vi "ble_read_specific_message.vi"(5 "Command Class (System)":T1 format="%02x" items=["System", "Persistent Store", "Attribute database", "Connection", "Attribute client", "Security Manager", "Generic Access Profile", "Hardware"], 6 "Stop if differnt to expected(F)":bool, 7 "Message Type (Response)":T2 format="%02x" items=["Command / Response"=0, "Event"=128], 8 "error in (no error)":errorcluster, 10 "Message ID (0x00)":u8 format="%02x", 11 "COM Bluegiga in":refnum<visa-resource-name>) -> (0 "error out":errorcluster, 1 "full message package":u8[](array[numeric]) format="%02x", 2 "specific payload":u8[](array[numeric]) format="%02x", 3 "COM Bluegiga out":refnum<visa-resource-name>, 4 "success?":bool)   [LabVIEW 2013]
uses:
  type_def/message_type.ctl
  type_def/message_class.ctl
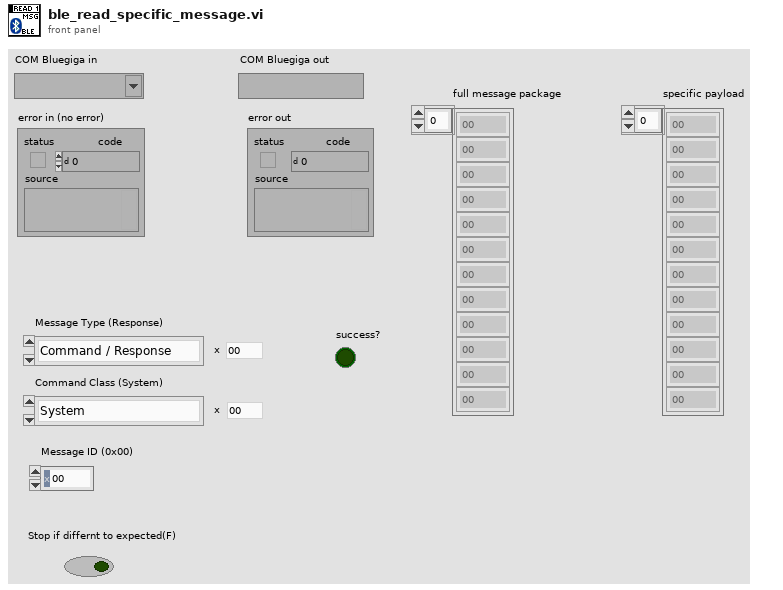
[diagram p1: front panel]
types:
  T1 = typedef "message_class.ctl" = u8
  T2 = typedef "message_type.ctl" = u8
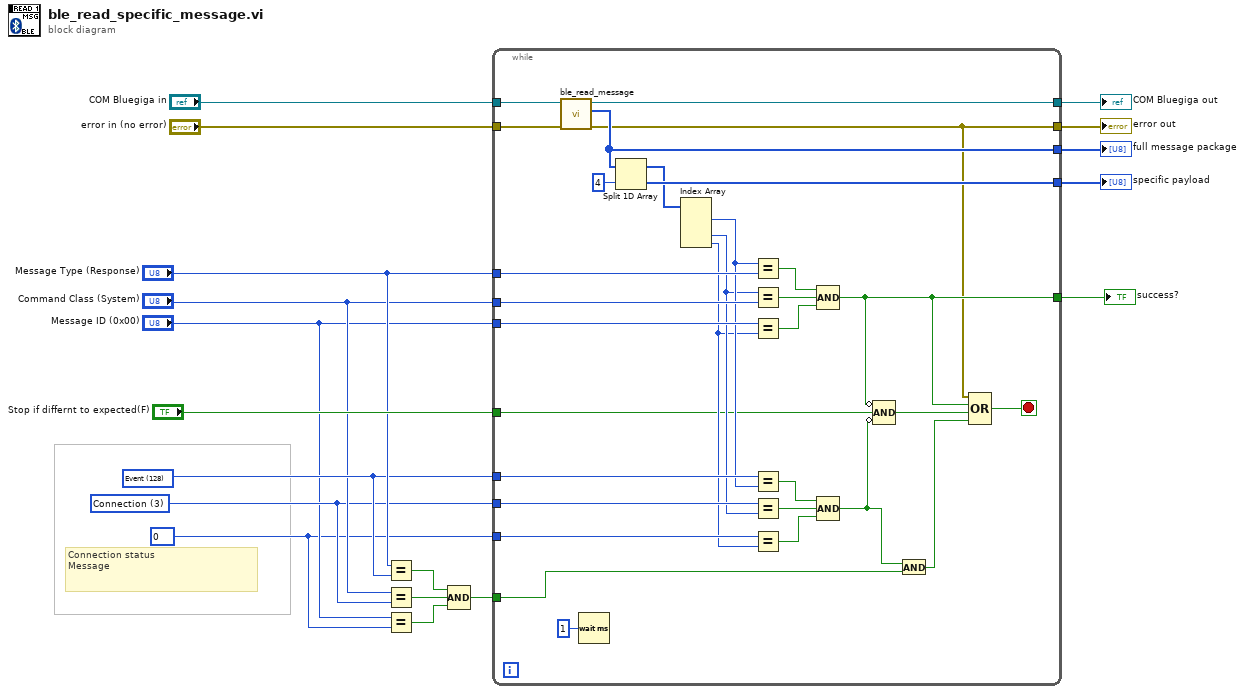
[diagram p0: block diagram]
diagram:
  w5 = u8 0 ("Message ID (0x00)")
  w7 = T1 3 items=["System", "Persistent Store", "Attribute database", "Connection", "Attribute client", "Security Manager", "Generic Access Profile", "Hardware"] ("Command Class (System)")
  w9 = T2 128 items=["Command / Response"=0, "Event"=128] ("Message Type (Response)")
  # "Connection status\nMessage"
  n1 = Equal?(x="Message Type (Response)", y=w9) -> (x = y?=w4:bool)
  n2 = Equal?(x="Command Class (System)", y=w7) -> (x = y?=w3:bool)
  n3 = Equal?(x="Message ID (0x00)", y=w5) -> (x = y?=w2:bool)
  n4 = Compound Arithmetic op=AND(w4, w3, w2) -> (w1:bool)
  n5 = while {
    tunnel: "COM Bluegiga in" -> [w49]
    tunnel: "error in (no error)" -> [w48]
    tunnel: [w47] -> w16
    tunnel: [w19] -> w15
    tunnel: "Message Type (Response)" -> [w46]
    tunnel: "Command Class (System)" -> [w45]
    tunnel: "Message ID (0x00)" -> [w44]
    tunnel: [w43] -> w14
    tunnel: [w42] -> w13
    tunnel: [w26] -> w12
    tunnel: w9 -> [w33]
    tunnel: w7 -> [w32]
    tunnel: w5 -> [w31]
    tunnel: "Stop if differnt to expected(F)" -> [w23]
    tunnel: w1 -> [w21]
    stop <- w22 stop-if-true
    n6 = call "ble_read_message.vi"("error in (no error)"=w48, "COM Bluegiga in"=w49) -> ("error out"=w19:errorcluster, "message package"=w43:u8[], "COM Bluegiga out"=w47:refnum<visa-resource-name>)  [unwired: 7 in]
    n7 = Wait (ms)(milliseconds to wait=u32 1) -> ()  [unwired: 1 out]
    n8 = Split 1D Array(array=w43, index=4) -> (first subarray=w40:u8[], second subarray=w42:u8[])
    n9 = Index Array(array=w40) -> (element #1=w30:u8, element #3=w29:u8, element #4=w28:u8)  [unwired: 4 in, 1 out]
    n10 = Equal?(x=w30, y=w46) -> (x = y?=w39:bool)
    n11 = Equal?(x=w29, y=w45) -> (x = y?=w38:bool)
    n12 = Equal?(x=w44, y=w28) -> (x = y?=w37:bool)
    n13 = Equal?(x=w33, y=w30) -> (x = y?=w34:bool)
    n14 = Equal?(x=w32, y=w29) -> (x = y?=w35:bool)
    n15 = Equal?(x=w31, y=w28) -> (x = y?=w36:bool)
    n16 = Compound Arithmetic op=AND(w39, w38, w37) -> (w26:bool)
    n17 = Compound Arithmetic op=AND(w34, w35, w36) -> (w24:bool)
    n18 = Compound Arithmetic op=AND(invert w26, w23, invert w24) -> (w25:bool)
    n19 = And(x=w24, y=w21) -> (x .and. y?=w27:bool)
    n20 = Compound Arithmetic op=OR(w19, w26, w25, w27) -> (w22:bool)
  }
  "COM Bluegiga out" <- w16
  "error out" <- w15
  "full message package" <- w14
  "specific payload" <- w13
  "success?" <- w12
